vi "Autonomous Independent.vi"   [LabVIEW 2019]
doc: "This VI is called when autonomous begins, and will automatically be terminated when autonomous ends. You can carry out timed or sensor driven robot movement independently without needing to return to the caller."
uses:
  <vilib>/Rock Robotics/WPI/Utilities/WPI_GetSetVariantRefNum.vi
  <vilib>/Rock Robotics/Network Tables/NT Write Numeric Array.vi
  <vilib>/addons/control/pid/NI_PID_pid.lvlib
  <vilib>/Rock Robotics/WPI/SafetyOutput/WPI_SafetyOutputConfigMenu.ctl
  <vilib>/addons/control/pid/pid.llb/PID (DBL).vi
types:
  T1 = typedef "WPI_SafetyOutputConfigMenu.ctl" = enum16{"Enable", "Disable"}
  T2 = typedef "WPI_JoystickDevRef.ctl" = cluster{"Device":T3}
  T3 = typedef "WPI_JoystickDeviceEnum.ctl" = enum16{"USB 0", "USB 1", "USB 2", "USB 3", "USB 4", "USB 5"}
  T4 = typedef "WPI_MotorControlDeviceRef.ctl" = cluster{"DeviceStatus":errorcluster, "Type":T5, "PWM":cluster{"PWM Channel":T6, "DeadBand":T7}, "CAN":cluster{"Device Number":u8, "SetOutput VI Ref":variant, "GetOutput VI Ref":variant, "Enable VI Ref":variant, "Disable VI Ref":variant, "Data":variant}, "Invert":bool, "DIO PWM":cluster{"PWM \"Enable\" Channel":T6, "DIOChannel":T8, "PWM Rate":dbl}}
  T5 = typedef "WPI_MotorControlType.ctl" = enum16{"PWM", "CAN", "DIO PWM"}
  T6 = typedef "FPGA_DIOPWMChannel.ctl" = enum8{"PWM 0", "PWM 1", "PWM 2", "PWM 3", "PWM 4", "PWM 5", "PWM 6", "PWM 7", "PWM 8", "PWM 9", "PWM MXP 0", "PWM MXP 1", "PWM MXP 2", "PWM MXP 3", "PWM MXP 4", "PWM MXP 5", "PWM MXP 6", "PWM MXP 7", "PWM MXP 8", "PWM MXP 9", "Invalid"}
  T7 = typedef "WPI_PWMDeadband.ctl" = cluster{"Name":string, "maxPositivePwm":i32, "minPositivePwm":i32, "centerPwm":i32, "maxNegativePwm":i32, "minNegativePwm":i32, "angularRange":u16}
  T8 = typedef "FPGA_DIOChannel.ctl" = enum8{"DIO 0", "DIO 1", "DIO 2", "DIO 3", "DIO 4", "DIO 5", "DIO 6", "DIO 7", "DIO 8", "DIO 9", "DIO MXP 0", "DIO MXP 1", "DIO MXP 2", "DIO MXP 3", "DIO MXP 4", "DIO MXP 5", "DIO MXP 6", "DIO MXP 7", "DIO MXP 8", "DIO MXP 9", "DIO MXP 10", "DIO MXP 11", "DIO MXP 12", "DIO MXP 13", "DIO MXP 14", "DIO MXP 15", "SPI Port CS1", "SPI Port CS2", "SPI Port CS3", "SPI Port MISO", "SPI Port MOSI", "Invalid"}
  T9 = typedef "WPI_DigitalInputDevRef.ctl" = cluster{"DevStatus":errorcluster, "DIO Channel":T8}
  T10 = cluster{"proportional gain (Kc)":dbl, "integral time (Ti, min)":dbl, "derivative time (Td, min)":dbl}
  T11 = cluster{"Yaw":dbl, "Roll":dbl, "Pitch":dbl, "Heading":dbl, "Fused Heading":dbl}
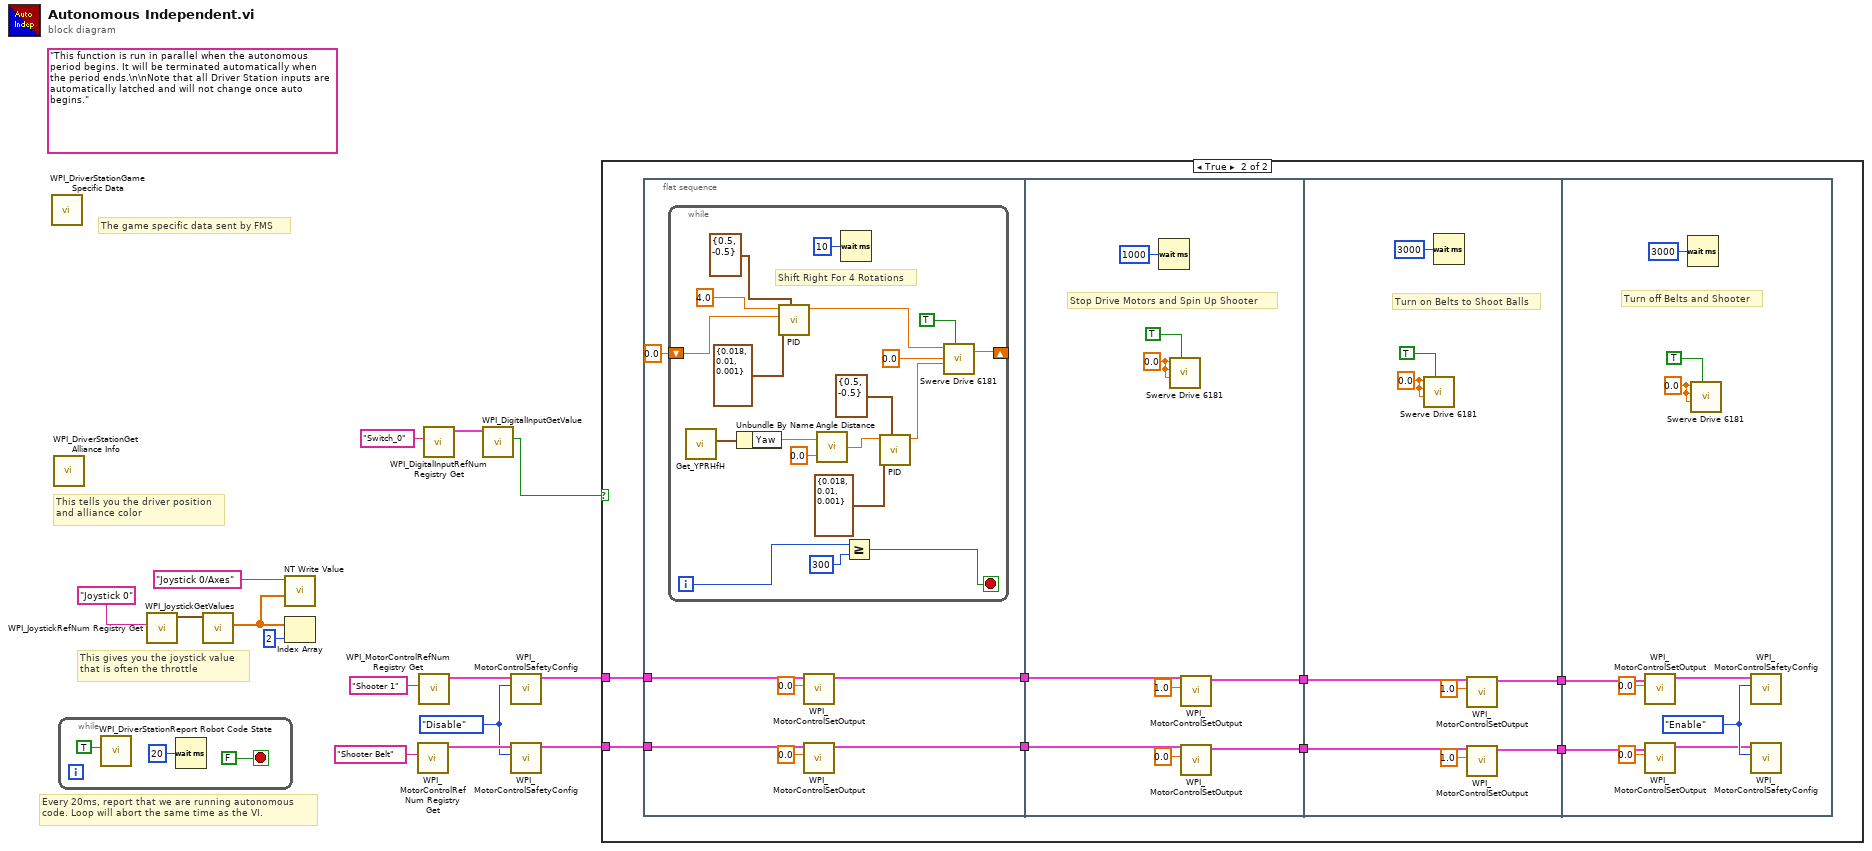
[diagram p0: block diagram]
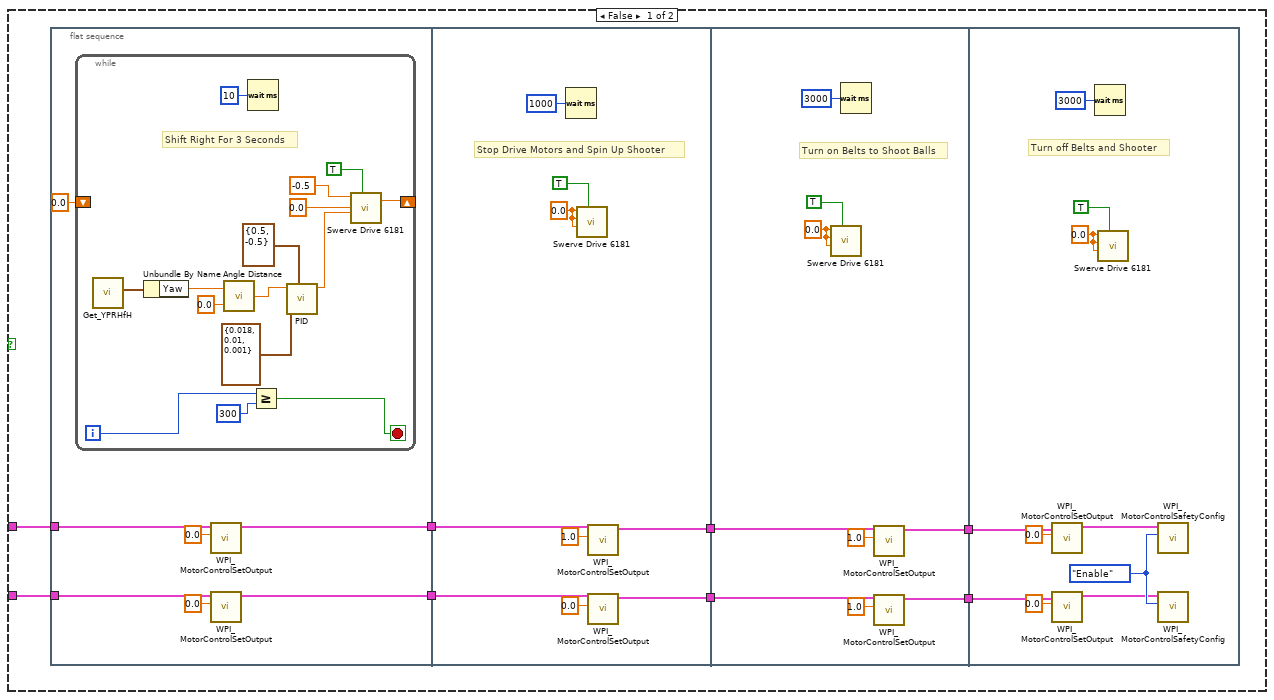
[diagram p2: hidden frame]
diagram:
  w6 = WPI_SafetyOutputConfigMenu."Disable" ("mode")
  (unwired) "This function is run in parallel when the autonomous period begins. It will be terminated automatically when the period ends.\n\nNote that all Driver Station inputs are automatically latched and will not change once auto begins."
  # "The game specific data sent by FMS"
  # "Every 20ms, report that we are running autonomous\ncode. Loop will abort the same time as the VI."
  # "This gives you the joystick value\nthat is often the throttle"
  # "This tells you the driver position\nand alliance color"
  n1 = call <vilib>:"WPI_DriverStationGame Specific Data.vi"() -> ()  [unwired: 11 in, 1 out]
  n2 = call <vilib>:"WPI_DriverStationGet Alliance Info.vi"() -> ()  [unwired: 12 out]
  n3 = while {
    stop <- FALSE stop-if-true
    n4 = call <vilib>:"WPI_DriverStationReport Robot Code State.vi"("Autonomous"=TRUE) -> ()  [unwired: 10 in, 1 out]
    n5 = Wait (ms)(milliseconds to wait=u32 20) -> ()  [unwired: 1 out]
  }
  n6 = call <vilib>:"WPI_JoystickRefNum Registry Get.vi"("refnum name"="Joystick 0") -> ("JoystickDevRef"=w14:T2)  [unwired: 1 in, 9 out]
  n7 = call <vilib>:"WPI_JoystickGetValues.vi"("JoystickDevRef"=w14) -> ("Axes"=w12:dbl[])  [unwired: 6 in, 4 out]
  n8 = call-poly <vilib>:"NT Write Value.vi"("Numeric Array"=w12, "Name"="Joystick 0/Axes") -> ()  [unwired: 9 in, 1 out]
  n9 = Index Array(array=w12, index=2) -> ()  [unwired: 1 out]
  n10 = call <vilib>:"WPI_MotorControlRefNum Registry Get.vi"("refnum name"="Shooter Belt") -> ("MotorControlDevRef"=w8:T4)  [unwired: 9 in, 1 out]
  n11 = call <vilib>:"WPI_MotorControlRefNum Registry Get.vi"("refnum name"="Shooter 1") -> ("MotorControlDevRef"=w7:T4)  [unwired: 9 in, 1 out]
  n12 = call <vilib>:"WPI_DigitalInputRefNum Registry Get.vi"("refnum name"="Switch_0") -> ("DigitalInputDevRef"=w3:T9)  [unwired: 9 in, 1 out]
  n13 = call <vilib>:"WPI_DigitalInputGetValue.vi"("DigitalInputDevRef"=w3) -> ("Value"=w2:bool)  [unwired: 8 in, 2 out]
  n14 = call <vilib>:"WPI_MotorControlSafetyConfig.vi"("mode"=w6, "MotorControlDevRef"=w7) -> ("MotorControlDevRef"=w4:T4)  [unwired: 8 in, 1 out]
  n15 = call <vilib>:"WPI_MotorControlSafetyConfig.vi"("mode"=w6, "MotorControlDevRef"=w8) -> ("MotorControlDevRef"=w5:T4)  [unwired: 8 in, 1 out]
  n16 = case shown="True" w2 {
    tunnel: w5 -> [w20 w78]
    tunnel: w4 -> [w19 w77]
    frame False {
      n17 = flat-sequence {
        tunnel: w20 -> [w33]
        tunnel: w19 -> [w32]
        tunnel: [w29] -> w26
        tunnel: [w28] -> w25
        tunnel: w26 -> [w54]
        tunnel: w25 -> [w53]
        tunnel: [w52] -> w24
        tunnel: [w51] -> w23
        tunnel: w24 -> [w65]
        tunnel: w23 -> [w64]
        tunnel: [w63] -> w22
        tunnel: [w62] -> w21
        tunnel: w22 -> [w75]
        tunnel: w21 -> [w74]
        frame #0 {
          n18 = while {
            shift-right: [w34] -> _
            shift-left: 0.0 ("Avg Sensor Pos") -> [_]
            i -> [w47]
            stop <- w46 stop-if-true
            # "Shift Right For 3 Seconds"
            n19 = call <vilib>:"Get_YPRHfH.vi"() -> ("YRPHfH"=w43:T11)  [unwired: 11 in]
            n20 = Unbundle By Name(w43) -> ("Yaw"=w42:dbl)
            n21 = call "Angle Distance.vi"("target angle"=0.0, "current angle"=w42) -> ("distance"=w44:dbl)
            n22 = Wait (ms)(milliseconds to wait=u32 10) -> ()  [unwired: 1 out]
            n23 = Greater Or Equal?(x=w47, y=300) -> (x >= y?=w46:bool)
            n24 = call-poly <vilib>:"PID.vi"("output range"=cluster{"output high":dbl, "output low":dbl} {"output high"=0.5, "output low"=-0.5}, "PID gains"=T10 {"proportional gain (Kc)"=0.018, "integral time (Ti, min)"=0.01, "derivative time (Td, min)"=0.001}, "setpoint"=w44) -> ("output"=w40:dbl)  [unwired: 7 in, 1 out]
            n25 = call "Swerve Drive 6181.vi"("X"=-0.5, "Y"=0.0, "Z"=w40, "Auto Controls"=TRUE) -> ("Avg Sensor Pos"=w34:dbl)  [unwired: 2 in]
          }
          n26 = call <vilib>:"WPI_MotorControlSetOutput.vi"("Output"=0.0, "MotorControlDevRef"=w32) -> ("MotorControlDevRef"=w29:T4)  [unwired: 7 in, 2 out]
          n27 = call <vilib>:"WPI_MotorControlSetOutput.vi"("Output"=0.0, "MotorControlDevRef"=w33) -> ("MotorControlDevRef"=w28:T4)  [unwired: 7 in, 2 out]
        }
        frame #1 {
          w56 = 0.0 ("X")
          # "Stop Drive Motors and Spin Up Shooter"
          n28 = Wait (ms)(milliseconds to wait=u32 1000) -> ()  [unwired: 1 out]
          n29 = call "Swerve Drive 6181.vi"("X"=w56, "Y"=w56, "Z"=w56, "Auto Controls"=TRUE) -> ()  [unwired: 2 in, 1 out]
          n30 = call <vilib>:"WPI_MotorControlSetOutput.vi"("Output"=1.0, "MotorControlDevRef"=w54) -> ("MotorControlDevRef"=w52:T4)  [unwired: 7 in, 2 out]
          n31 = call <vilib>:"WPI_MotorControlSetOutput.vi"("Output"=0.0, "MotorControlDevRef"=w53) -> ("MotorControlDevRef"=w51:T4)  [unwired: 7 in, 2 out]
        }
        frame #2 {
          w59 = 0.0 ("X")
          # "Turn on Belts to Shoot Balls"
          n32 = call "Swerve Drive 6181.vi"("X"=w59, "Y"=w59, "Z"=w59, "Auto Controls"=TRUE) -> ()  [unwired: 2 in, 1 out]
          n33 = Wait (ms)(milliseconds to wait=u32 3000) -> ()  [unwired: 1 out]
          n34 = call <vilib>:"WPI_MotorControlSetOutput.vi"("Output"=1.0, "MotorControlDevRef"=w65) -> ("MotorControlDevRef"=w63:T4)  [unwired: 7 in, 2 out]
          n35 = call <vilib>:"WPI_MotorControlSetOutput.vi"("Output"=1.0, "MotorControlDevRef"=w64) -> ("MotorControlDevRef"=w62:T4)  [unwired: 7 in, 2 out]
        }
        frame #3 {
          w67 = 0.0 ("X")
          w71 = WPI_SafetyOutputConfigMenu."Enable" ("mode")
          # "Turn off Belts and Shooter"
          n36 = call <vilib>:"WPI_MotorControlSetOutput.vi"("Output"=0.0, "MotorControlDevRef"=w75) -> ("MotorControlDevRef"=w70:T4)  [unwired: 7 in, 2 out]
          n37 = call <vilib>:"WPI_MotorControlSetOutput.vi"("Output"=0.0, "MotorControlDevRef"=w74) -> ("MotorControlDevRef"=w69:T4)  [unwired: 7 in, 2 out]
          n38 = Wait (ms)(milliseconds to wait=u32 3000) -> ()  [unwired: 1 out]
          n39 = call "Swerve Drive 6181.vi"("X"=w67, "Y"=w67, "Z"=w67, "Auto Controls"=TRUE) -> ()  [unwired: 2 in, 1 out]
          n40 = call <vilib>:"WPI_MotorControlSafetyConfig.vi"("mode"=w71, "MotorControlDevRef"=w70) -> ()  [unwired: 8 in, 2 out]
          n41 = call <vilib>:"WPI_MotorControlSafetyConfig.vi"("mode"=w71, "MotorControlDevRef"=w69) -> ()  [unwired: 8 in, 2 out]
        }
      }
    }
    frame True {
      n42 = flat-sequence {
        tunnel: w78 -> [w91]
        tunnel: w77 -> [w90]
        tunnel: [w87] -> w84
        tunnel: [w86] -> w83
        tunnel: w84 -> [w116]
        tunnel: w83 -> [w115]
        tunnel: [w114] -> w82
        tunnel: [w113] -> w81
        tunnel: w82 -> [w127]
        tunnel: w81 -> [w126]
        tunnel: [w125] -> w80
        tunnel: [w124] -> w79
        tunnel: w80 -> [w137]
        tunnel: w79 -> [w136]
        frame #0 {
          n43 = while {
            shift-right: [w98] -> _
            shift-left: 0.0 ("Avg Sensor Pos") -> [w93]
            i -> [w109]
            stop <- w108 stop-if-true
            # "Shift Right For 4 Rotations"
            n44 = call <vilib>:"Get_YPRHfH.vi"() -> ("YRPHfH"=w105:T11)  [unwired: 11 in]
            n45 = Unbundle By Name(w105) -> ("Yaw"=w104:dbl)
            n46 = call-poly <vilib>:"PID.vi"("output range"=cluster{"output high":dbl, "output low":dbl} {"output high"=0.5, "output low"=-0.5}, "PID gains"=T10 {"proportional gain (Kc)"=0.018, "integral time (Ti, min)"=0.01, "derivative time (Td, min)"=0.001}, "process variable"=w93, "setpoint"=4.0) -> ("output"=w94:dbl)  [unwired: 6 in, 1 out]
            n47 = call "Angle Distance.vi"("target angle"=0.0, "current angle"=w104) -> ("distance"=w106:dbl)
            n48 = Wait (ms)(milliseconds to wait=u32 10) -> ()  [unwired: 1 out]
            n49 = Greater Or Equal?(x=w109, y=300) -> (x >= y?=w108:bool)
            n50 = call-poly <vilib>:"PID.vi"("output range"=cluster{"output high":dbl, "output low":dbl} {"output high"=0.5, "output low"=-0.5}, "PID gains"=T10 {"proportional gain (Kc)"=0.018, "integral time (Ti, min)"=0.01, "derivative time (Td, min)"=0.001}, "setpoint"=w106) -> ("output"=w102:dbl)  [unwired: 7 in, 1 out]
            n51 = call "Swerve Drive 6181.vi"("X"=w94, "Y"=0.0, "Z"=w102, "Auto Controls"=TRUE) -> ("Avg Sensor Pos"=w98:dbl)  [unwired: 2 in]
          }
          n52 = call <vilib>:"WPI_MotorControlSetOutput.vi"("Output"=0.0, "MotorControlDevRef"=w90) -> ("MotorControlDevRef"=w87:T4)  [unwired: 7 in, 2 out]
          n53 = call <vilib>:"WPI_MotorControlSetOutput.vi"("Output"=0.0, "MotorControlDevRef"=w91) -> ("MotorControlDevRef"=w86:T4)  [unwired: 7 in, 2 out]
        }
        frame #1 {
          w118 = 0.0 ("X")
          # "Stop Drive Motors and Spin Up Shooter"
          n54 = Wait (ms)(milliseconds to wait=u32 1000) -> ()  [unwired: 1 out]
          n55 = call "Swerve Drive 6181.vi"("X"=w118, "Y"=w118, "Z"=w118, "Auto Controls"=TRUE) -> ()  [unwired: 2 in, 1 out]
          n56 = call <vilib>:"WPI_MotorControlSetOutput.vi"("Output"=1.0, "MotorControlDevRef"=w116) -> ("MotorControlDevRef"=w114:T4)  [unwired: 7 in, 2 out]
          n57 = call <vilib>:"WPI_MotorControlSetOutput.vi"("Output"=0.0, "MotorControlDevRef"=w115) -> ("MotorControlDevRef"=w113:T4)  [unwired: 7 in, 2 out]
        }
        frame #2 {
          w121 = 0.0 ("X")
          # "Turn on Belts to Shoot Balls"
          n58 = call "Swerve Drive 6181.vi"("X"=w121, "Y"=w121, "Z"=w121, "Auto Controls"=TRUE) -> ()  [unwired: 2 in, 1 out]
          n59 = Wait (ms)(milliseconds to wait=u32 3000) -> ()  [unwired: 1 out]
          n60 = call <vilib>:"WPI_MotorControlSetOutput.vi"("Output"=1.0, "MotorControlDevRef"=w127) -> ("MotorControlDevRef"=w125:T4)  [unwired: 7 in, 2 out]
          n61 = call <vilib>:"WPI_MotorControlSetOutput.vi"("Output"=1.0, "MotorControlDevRef"=w126) -> ("MotorControlDevRef"=w124:T4)  [unwired: 7 in, 2 out]
        }
        frame #3 {
          w129 = 0.0 ("X")
          w133 = WPI_SafetyOutputConfigMenu."Enable" ("mode")
          # "Turn off Belts and Shooter"
          n62 = call <vilib>:"WPI_MotorControlSetOutput.vi"("Output"=0.0, "MotorControlDevRef"=w137) -> ("MotorControlDevRef"=w132:T4)  [unwired: 7 in, 2 out]
          n63 = call <vilib>:"WPI_MotorControlSetOutput.vi"("Output"=0.0, "MotorControlDevRef"=w136) -> ("MotorControlDevRef"=w131:T4)  [unwired: 7 in, 2 out]
          n64 = Wait (ms)(milliseconds to wait=u32 3000) -> ()  [unwired: 1 out]
          n65 = call "Swerve Drive 6181.vi"("X"=w129, "Y"=w129, "Z"=w129, "Auto Controls"=TRUE) -> ()  [unwired: 2 in, 1 out]
          n66 = call <vilib>:"WPI_MotorControlSafetyConfig.vi"("mode"=w133, "MotorControlDevRef"=w132) -> ()  [unwired: 8 in, 2 out]
          n67 = call <vilib>:"WPI_MotorControlSafetyConfig.vi"("mode"=w133, "MotorControlDevRef"=w131) -> ()  [unwired: 8 in, 2 out]
        }
      }
    }
  }
